vi "GetStrFromDigitalCtrl.vi"(10 "정밀도":u8, 11 "double ref":refnum<vi>) -> (3 "result":string)   [LabVIEW 2018, in "Library-Ctrl.lvlib"]
uses:
  Library-Ctrl.lvlib
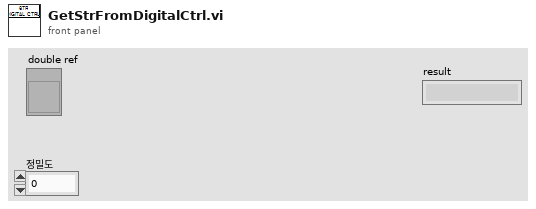
[diagram p1: front panel]
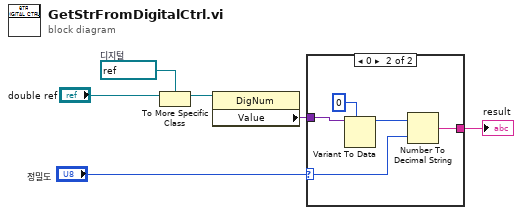
[diagram p0: block diagram]
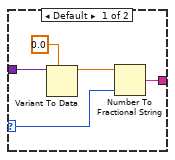
[diagram p2: hidden frame]
diagram:
  w5 = refnum<vi> refnum  # 디지털
  n1 = To More Specific Class(target class=w5, reference="double ref") -> (specific class reference=w4:refnum<vi>)  [unwired: 1 in, 1 out]
  n2 = property class="DigNum"(reference=w4) -> ("Value"=w3:variant)  [unwired: 1 in, 2 out]
  n3 = case shown="0" "정밀도" {
    selector: "정밀도" -> [w7 w12]
    tunnel: w3 -> [w11 w16]
    tunnel: [w8 w13] -> w2
    frame Default {
      n4 = Variant To Data(type=0.0, Variant=w11) -> (data=w9:dbl)  [unwired: 1 in, 1 out]
      n5 = Number To Fractional String(number=w9, precision (6)=w7) -> (F-format string=w8:string)  [unwired: 2 in]
    }
    frame 0 {
      n6 = Variant To Data(type=0, Variant=w16) -> (data=w14:i32)  [unwired: 1 in, 1 out]
      n7 = Number To Decimal String(number=w14, width (-)=w12) -> (decimal integer string=w13:string)
    }
  }
  "result" <- w2
